vi "_RT_CtrlLoop_WfmData_Gate.vi"(6 "ExpVar in":refnum<class "ExpVar.lvclass">, 8 "error in (no error)":errorcluster) -> ()   [LabVIEW 2018]
uses:
  PublicSubVI/NewExpVar/ExpVar.lvclass
  PublicSubVI/Ctl/_ctl_RT_NS_Status.ctl
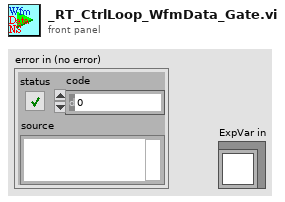
[diagram p1: front panel]
types:
  T1 = enum16{"via string label", "Laser", "Pressure", "TMP", "Script", "Signal Remarks", "ExtAO", "ExtDO", "ExtDI", "D999"}
  T2 = enum16{"None", "D999", "ExtAO", "ExtDO", "ExtDI_Label", "Signal_Remarks", "Script"}
  T3 = typedef "_ctl_RT_NS_Status.ctl" = enum8{"Idle", "Init", "Connected", "Stop"}
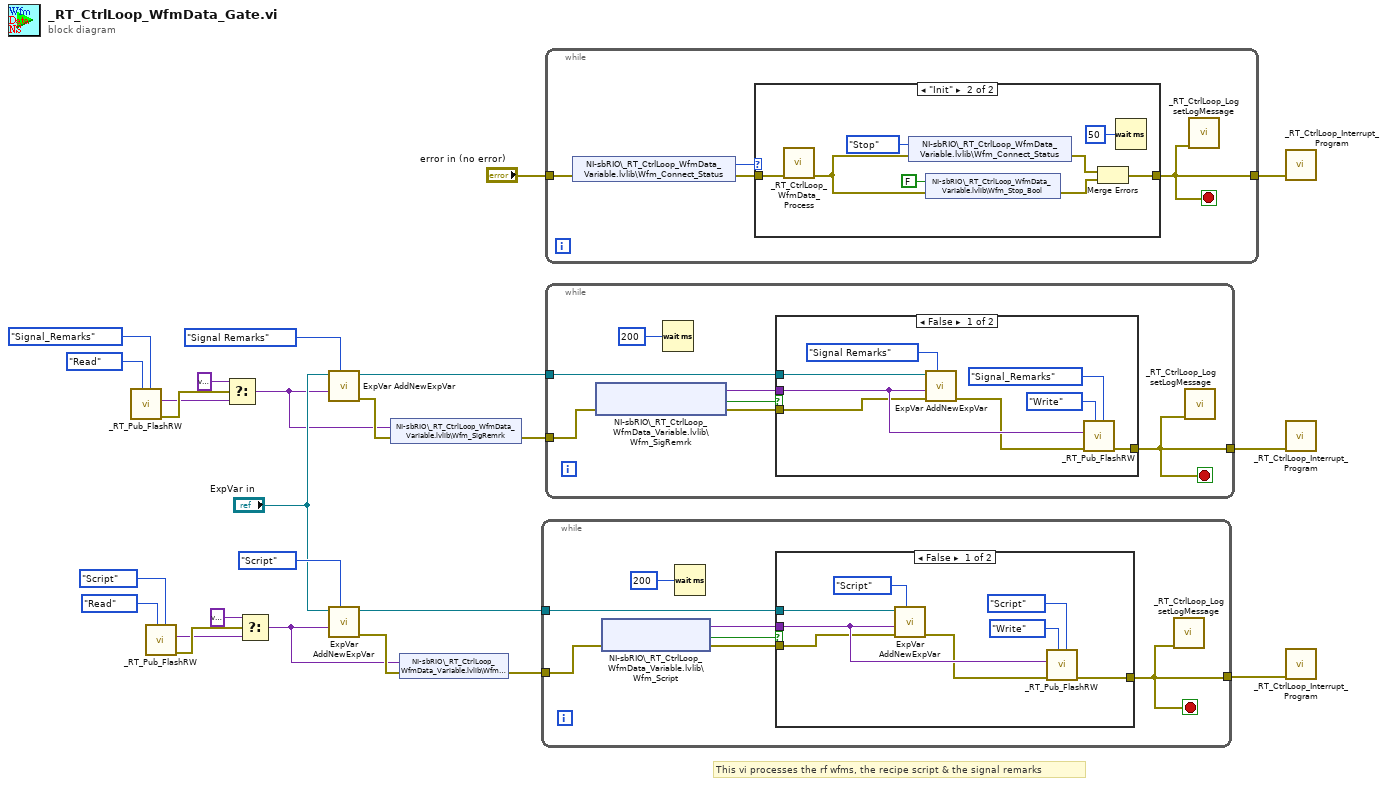
[diagram p0: block diagram]
diagram:
  # "This vi processes the rf wfms, the recipe script & the signal remarks"
  n1 = call "_RT_Pub_FlashRW.vi"("FileEnum"=T2."Signal_Remarks", "State"=enum16{"Read", "Write"}."Read") -> ("error out"=w3:errorcluster, "Value"=w2:variant)  [unwired: 7 in, 1 out]
  n2 = call "_RT_Pub_FlashRW.vi"("FileEnum"=T2."Script", "State"=enum16{"Read", "Write"}."Read") -> ("error out"=w8:errorcluster, "Value"=w7:variant)  [unwired: 7 in, 1 out]
  n3 = Select(t=variant, s=w3, f=w2) -> (s? t:f=w1:variant)
  n4 = Select(t=variant, s=w8, f=w7) -> (s? t:f=w5:variant)
  n5 = call-dynamic "ExpVar AddNewExpVar.vi"("VarType"=T1."Signal Remarks", "Var"=w1, "ExpVar in"="ExpVar in") -> ("error out"=w15:errorcluster, "NewExpVar out"=w18:refnum<class "ExpVar.lvclass">)  [unwired: 7 in]
  n6 = call-dynamic "ExpVar AddNewExpVar.vi"("VarType"=T1."Script", "Var"=w5, "ExpVar in"="ExpVar in") -> ("error out"=w13:errorcluster, "NewExpVar out"=w16:refnum<class "ExpVar.lvclass">)  [unwired: 7 in]
  n7 = shared-variable "NI-sbRIO\\_RT_CtrlLoop_WfmData_Variable.lvlib\\Wfm_SigRemrk"(w1, error in=w15) -> (error out=w14:errorcluster)
  n8 = shared-variable "NI-sbRIO\\_RT_CtrlLoop_WfmData_Variable.lvlib\\Wfm_Script"(w5, error in=w13) -> (error out=w12:errorcluster)
  n9 = while {
    tunnel: w16 -> [w32]
    tunnel: w12 -> [w27]
    tunnel: [w26] -> w9
    stop <- w26 stop-if-true
    n10 = shared-variable "NI-sbRIO\\_RT_CtrlLoop_WfmData_Variable.lvlib\\Wfm_Script"(error in=w27) -> (w30:variant, error out=w28:errorcluster, w29:bool)  [unwired: 1 in]
    n11 = Wait (ms)(milliseconds to wait=u32 200) -> ()  [unwired: 1 out]
    n12 = case shown="False" w29 {
      tunnel: w30 -> [w38 _]
      tunnel: w28 -> [w35 w41]
      tunnel: w32 -> [w40 _]
      tunnel: [w33 w41] -> w26
      frame False {
        n13 = call-dynamic "ExpVar AddNewExpVar.vi"("VarType"=T1."Script", "error in (no error)"=w35, "Var"=w38, "ExpVar in"=w40) -> ("error out"=w34:errorcluster)  [unwired: 6 in, 1 out]
        n14 = call "_RT_Pub_FlashRW.vi"("FileEnum"=T2."Script", "State"=enum16{"Read", "Write"}."Write", "error in (no error)"=w34, "DataIn"=w38) -> ("error out"=w33:errorcluster)  [unwired: 5 in, 2 out]
      }
      frame True {
      }
    }
    n15 = call "_RT_CtrlLoop_Log setLogMessage.vi"("error in"=w26) -> ()  [unwired: 9 in, 2 out]
  }
  n16 = while {
    tunnel: "error in (no error)" -> [w45]
    tunnel: [w42] -> w11
    stop <- w42 stop-if-true
    n17 = shared-variable "NI-sbRIO\\_RT_CtrlLoop_WfmData_Variable.lvlib\\Wfm_Connect_Status"(error in=w45) -> (w44:T3, error out=w43:errorcluster)
    n18 = case shown="\"Init\"" w44 {
      tunnel: w43 -> [w46 w54]
      tunnel: [w46 w51] -> w42
      frame "Stop", Default {
      }
      frame "Init" {
        n19 = call "_RT_CtrlLoop_WfmData_Process.vi"("error in (no error)"=w54) -> ("error out"=w47:errorcluster)  [unwired: 10 in]
        n20 = shared-variable "NI-sbRIO\\_RT_CtrlLoop_WfmData_Variable.lvlib\\Wfm_Connect_Status"(_ctl_RT_NS_Status."Stop" ("Wfm_Connect_Status"), error in=w47) -> (error out=w53:errorcluster)
        n21 = shared-variable "NI-sbRIO\\_RT_CtrlLoop_WfmData_Variable.lvlib\\Wfm_Stop_Bool"(FALSE ("Wfm_Stop_Bool"), error in=w47) -> (error out=w52:errorcluster)
        n22 = Merge Errors(w53, w52) -> (w51:errorcluster)
        n23 = Wait (ms)(milliseconds to wait=u32 50 ("millisecond multiple")) -> ()  [unwired: 1 out]
      }
    }
    n24 = call "_RT_CtrlLoop_Log setLogMessage.vi"("error in"=w42) -> ()  [unwired: 9 in, 2 out]
  }
  n25 = while {
    tunnel: w18 -> [w58]
    tunnel: w14 -> [w56]
    tunnel: [w55] -> w10
    stop <- w55 stop-if-true
    n26 = shared-variable "NI-sbRIO\\_RT_CtrlLoop_WfmData_Variable.lvlib\\Wfm_SigRemrk"(error in=w56) -> (w60:variant, error out=w59:errorcluster, w61:bool)  [unwired: 1 in]
    n27 = Wait (ms)(milliseconds to wait=u32 200) -> ()  [unwired: 1 out]
    n28 = case shown="False" w61 {
      tunnel: w60 -> [w67 _]
      tunnel: w59 -> [w64 w70]
      tunnel: w58 -> [w69 _]
      tunnel: [w62 w70] -> w55
      frame False {
        n29 = call-dynamic "ExpVar AddNewExpVar.vi"("VarType"=T1."Signal Remarks", "error in (no error)"=w64, "Var"=w67, "ExpVar in"=w69) -> ("error out"=w63:errorcluster)  [unwired: 6 in, 1 out]
        n30 = call "_RT_Pub_FlashRW.vi"("FileEnum"=T2."Signal_Remarks", "State"=enum16{"Read", "Write"}."Write", "error in (no error)"=w63, "DataIn"=w67) -> ("error out"=w62:errorcluster)  [unwired: 5 in, 2 out]
      }
      frame True {
      }
    }
    n31 = call "_RT_CtrlLoop_Log setLogMessage.vi"("error in"=w55) -> ()  [unwired: 9 in, 2 out]
  }
  n32 = call "_RT_CtrlLoop_Interrupt_Program.vi"("error in (no error)"=w11) -> ()  [unwired: 10 in, 1 out]
  n33 = call "_RT_CtrlLoop_Interrupt_Program.vi"("error in (no error)"=w10) -> ()  [unwired: 10 in, 1 out]
  n34 = call "_RT_CtrlLoop_Interrupt_Program.vi"("error in (no error)"=w9) -> ()  [unwired: 10 in, 1 out]
